vi "Periodic Tasks.vi"(8 "error in":errorcluster) -> ()   [LabVIEW 2018]
doc: "This VI runs in parallel to other tasks. It can contain as many user-defined periodic loops as you need. These can carry out PID or other sorts of timed response."
uses:
  <vilib>/Rock Robotics/WPI/Utilities/WPI_GetSetVariantRefNum.vi
  Robot Global Data.vi
panel:
  in  "PID Constants":T1={"proportional gain (Kc)"=1.0, "integral time (Ti, min)"=0.01, "derivative time (Td, min)"=0.0} {"derivative time (Td, min)" format="%.3f"; "integral time (Ti, min)" format="%.3f"; "proportional gain (Kc)" format="%.3f"}
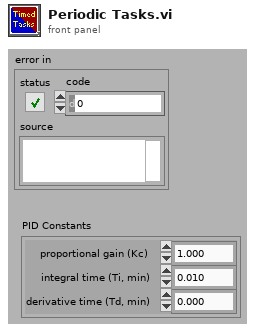
[diagram p1: front panel]
types:
  T1 = cluster{"proportional gain (Kc)":dbl, "integral time (Ti, min)":dbl, "derivative time (Td, min)":dbl}
  T2 = typedef "WPI_MotorControlDeviceRef.ctl" = cluster{"DeviceStatus":errorcluster, "Type":T3, "PWM":cluster{"PWM Channel":T4, "DeadBand":T5}, "CAN":cluster{"Device Number":u8, "SetOutput VI Ref":variant, "GetOutput VI Ref":variant, "Enable VI Ref":variant, "Disable VI Ref":variant, "Data":variant}, "Invert":bool, "DIO PWM":cluster{"PWM \"Enable\" Channel":T4, "DIOChannel":T6, "PWM Rate":dbl}}
  T3 = typedef "WPI_MotorControlType.ctl" = enum16{"PWM", "CAN", "DIO PWM"}
  T4 = typedef "FPGA_DIOPWMChannel.ctl" = enum8{"PWM 0", "PWM 1", "PWM 2", "PWM 3", "PWM 4", "PWM 5", "PWM 6", "PWM 7", "PWM 8", "PWM 9", "PWM MXP 0", "PWM MXP 1", "PWM MXP 2", "PWM MXP 3", "PWM MXP 4", "PWM MXP 5", "PWM MXP 6", "PWM MXP 7", "PWM MXP 8", "PWM MXP 9", "Invalid"}
  T5 = typedef "WPI_PWMDeadband.ctl" = cluster{"Name":string, "maxPositivePwm":i32, "minPositivePwm":i32, "centerPwm":i32, "maxNegativePwm":i32, "minNegativePwm":i32, "angularRange":u16}
  T6 = typedef "FPGA_DIOChannel.ctl" = enum8{"DIO 0", "DIO 1", "DIO 2", "DIO 3", "DIO 4", "DIO 5", "DIO 6", "DIO 7", "DIO 8", "DIO 9", "DIO MXP 0", "DIO MXP 1", "DIO MXP 2", "DIO MXP 3", "DIO MXP 4", "DIO MXP 5", "DIO MXP 6", "DIO MXP 7", "DIO MXP 8", "DIO MXP 9", "DIO MXP 10", "DIO MXP 11", "DIO MXP 12", "DIO MXP 13", "DIO MXP 14", "DIO MXP 15", "SPI Port CS1", "SPI Port CS2", "SPI Port CS3", "SPI Port MISO", "SPI Port MOSI", "Invalid"}
  T7 = typedef "WPI_JoystickDevRef.ctl" = cluster{"Device":T8}
  T8 = typedef "WPI_JoystickDeviceEnum.ctl" = enum16{"USB 0", "USB 1", "USB 2", "USB 3", "USB 4", "USB 5"}
  T9 = typedef "WPI_SolenoidDevRef.ctl" = cluster{"DevStatus":errorcluster, "Pneumatics Control Module":u8, "Forward Solenoid Channel":T10, "Reverse Solenoid Channel":T10}
  T10 = typedef "WPI_SolenoidChannel.ctl" = enum8{"Solenoid 0", "Solenoid 1", "Solenoid 2", "Solenoid 3", "Solenoid 4", "Solenoid 5", "Solenoid 6", "Solenoid 7", "Invalid"}
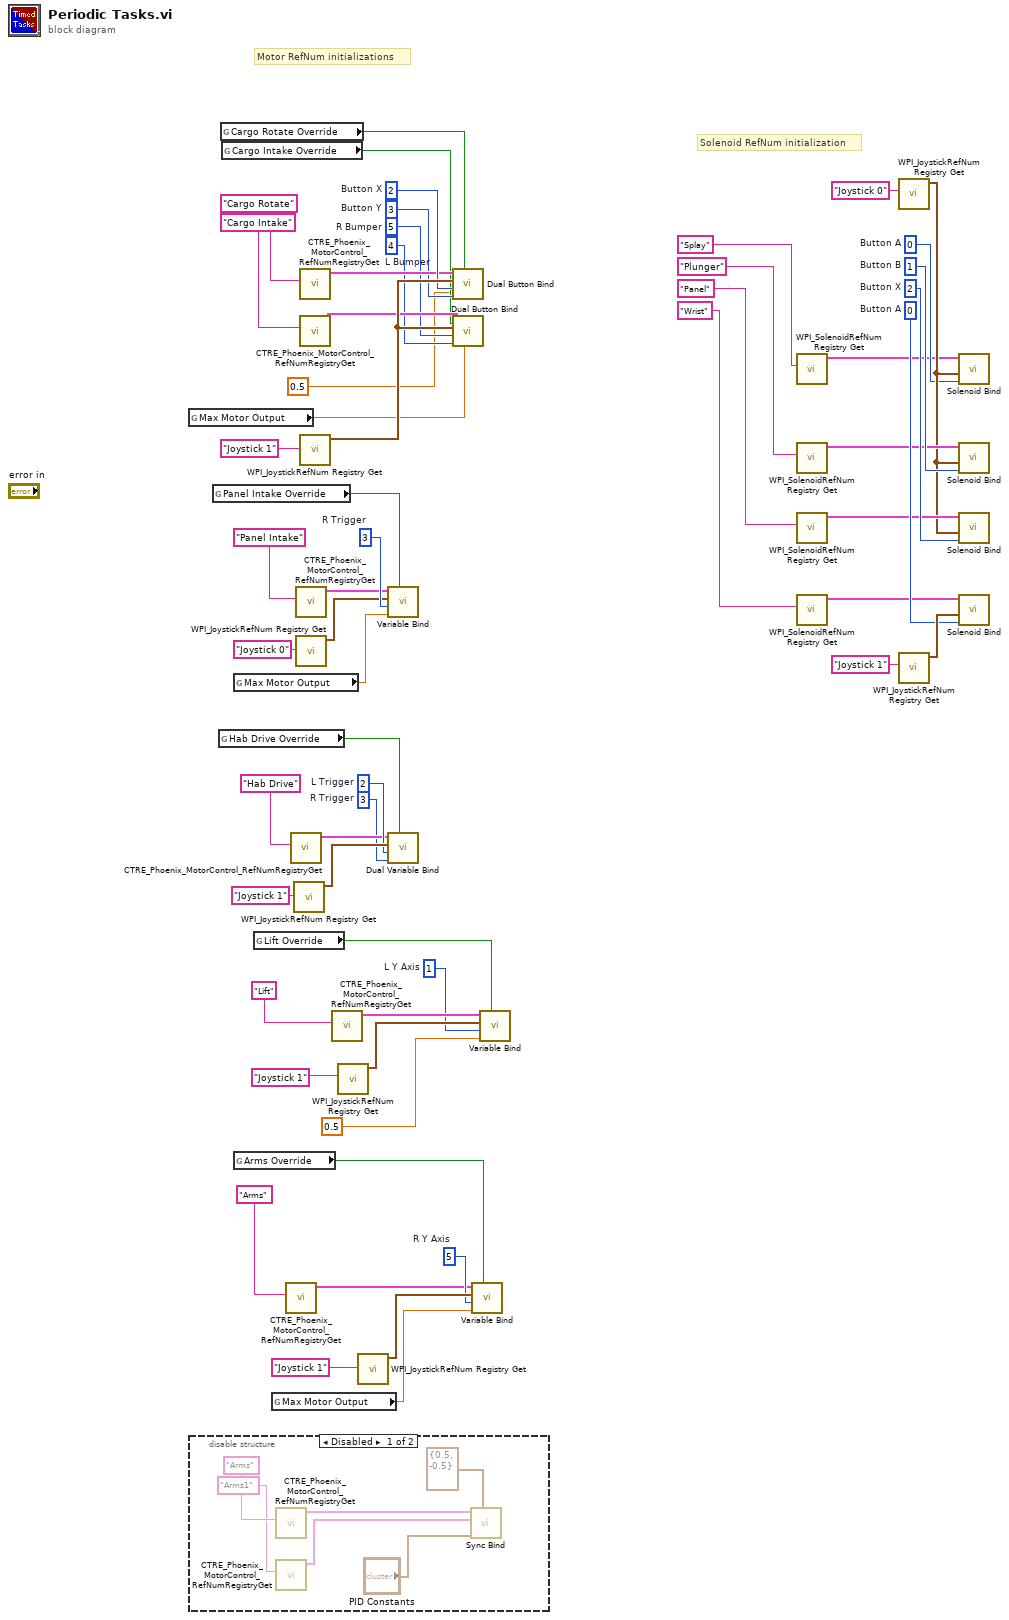
[diagram p0: block diagram]
diagram:
  w32 = 0  # Button A
  w34 = 2  # Button X
  w33 = 1  # Button B
  w27 = 0  # Button A
  w56 = 5  # R Y Axis
  w10 = 1  # L Y Axis
  w13 = 3  # R Trigger
  w50 = 2  # L Trigger
  w49 = 3  # R Trigger
  w14 = 4  # L Bumper
  w16 = 3  # Button Y
  w15 = 5  # R Bumper
  w43 = 2  # Button X
  # "Solenoid RefNum initialization"
  # "Motor RefNum initializations"
  n1 = global read "Robot Global Data.vi" "Max Motor Output"() -> (w2:dbl)
  n2 = disable-structure shown="Disabled" {
    frame Disabled {
      n3 = call <vilib>:"CTRE_Phoenix_MotorControl_RefNumRegistryGet.vi"("refnum name"="Arms") -> ("PhoenixMotorControlDevRef"=w62:T2)  [unwired: 9 in, 1 out]
      n4 = call <vilib>:"CTRE_Phoenix_MotorControl_RefNumRegistryGet.vi"("refnum name"="Arms1") -> ("PhoenixMotorControlDevRef"=w61:T2)  [unwired: 9 in, 1 out]
      n5 = call "Sync Bind.vi"("output range"=cluster{"output high":dbl, "output low":dbl} {"output high"=0.5, "output low"=-0.5}, "PID Constants"="PID Constants", "SlaveDevRef"=w61, "MasterDevRef"=w62) -> ()  [unwired: 8 in]
    }
    frame Enabled {
    }
  }
  n6 = global read "Robot Global Data.vi" "Panel Intake Override"() -> (w7:bool)
  n7 = global read "Robot Global Data.vi" "Hab Drive Override"() -> (w6:bool)
  n8 = global read "Robot Global Data.vi" "Cargo Rotate Override"() -> (w9:bool)
  n9 = global read "Robot Global Data.vi" "Cargo Intake Override"() -> (w8:bool)
  n10 = global read "Robot Global Data.vi" "Max Motor Output"() -> (w54:dbl)
  n11 = global read "Robot Global Data.vi" "Arms Override"() -> (w4:bool)
  n12 = global read "Robot Global Data.vi" "Lift Override"() -> (w5:bool)
  n13 = global read "Robot Global Data.vi" "Max Motor Output"() -> (w55:dbl)
  n14 = call <vilib>:"CTRE_Phoenix_MotorControl_RefNumRegistryGet.vi"("refnum name"="Arms") -> ("PhoenixMotorControlDevRef"=w20:T2)  [unwired: 9 in, 1 out]
  n15 = call <vilib>:"CTRE_Phoenix_MotorControl_RefNumRegistryGet.vi"("refnum name"="Hab Drive") -> ("PhoenixMotorControlDevRef"=w19:T2)  [unwired: 9 in, 1 out]
  n16 = call <vilib>:"WPI_JoystickRefNum Registry Get.vi"("refnum name"="Joystick 1") -> ("JoystickDevRef"=w52:T7)  [unwired: 9 in, 1 out]
  n17 = call <vilib>:"CTRE_Phoenix_MotorControl_RefNumRegistryGet.vi"("refnum name"="Panel Intake") -> ("PhoenixMotorControlDevRef"=w47:T2)  [unwired: 9 in, 1 out]
  n18 = call <vilib>:"WPI_JoystickRefNum Registry Get.vi"("refnum name"="Joystick 0") -> ("JoystickDevRef"=w48:T7)  [unwired: 9 in, 1 out]
  n19 = call <vilib>:"CTRE_Phoenix_MotorControl_RefNumRegistryGet.vi"("refnum name"="Cargo Rotate") -> ("PhoenixMotorControlDevRef"=w18:T2)  [unwired: 9 in, 1 out]
  n20 = call <vilib>:"CTRE_Phoenix_MotorControl_RefNumRegistryGet.vi"("refnum name"="Cargo Intake") -> ("PhoenixMotorControlDevRef"=w17:T2)  [unwired: 9 in, 1 out]
  n21 = call <vilib>:"WPI_JoystickRefNum Registry Get.vi"("refnum name"="Joystick 1") -> ("JoystickDevRef"=w45:T7)  [unwired: 9 in, 1 out]
  n22 = call <vilib>:"CTRE_Phoenix_MotorControl_RefNumRegistryGet.vi"("refnum name"="Lift") -> ("PhoenixMotorControlDevRef"=w12:T2)  [unwired: 9 in, 1 out]
  n23 = call <vilib>:"WPI_JoystickRefNum Registry Get.vi"("refnum name"="Joystick 1") -> ("JoystickDevRef"=w11:T7)  [unwired: 9 in, 1 out]
  n24 = call <vilib>:"WPI_JoystickRefNum Registry Get.vi"("refnum name"="Joystick 1") -> ("JoystickDevRef"=w57:T7)  [unwired: 9 in, 1 out]
  n25 = call "Variable Bind.vi"("Override"=w7, "Ouput"=w54, "Axis ID"=w49, "JoystickDevRef"=w48, "PhoenixMotorControlDevRef"=w47) -> ()  [unwired: 6 in, 1 out]
  n26 = call "Dual Variable Bind.vi"("Override"=w6, "Reverse ID"=w13, "Forward ID"=w50, "JoystickDevRef"=w52, "PhoenixMotorControlDevRef"=w19) -> ()  [unwired: 6 in, 1 out]
  n27 = call "Dual Button Bind.vi"("Output"=0.5, "Override"=w9, "Reverse ID"=w16, "Forward ID"=w43, "JoystickDevRef"=w45, "PhoenixMotorControlDevRef"=w18) -> ()  [unwired: 5 in, 1 out]
  n28 = call "Dual Button Bind.vi"("Output"=w2, "Override"=w8, "Reverse ID"=w14, "Forward ID"=w15, "JoystickDevRef"=w45, "PhoenixMotorControlDevRef"=w17) -> ()  [unwired: 5 in, 1 out]
  n29 = call "Variable Bind.vi"("Override"=w4, "Ouput"=w55, "Axis ID"=w56, "JoystickDevRef"=w57, "PhoenixMotorControlDevRef"=w20) -> ()  [unwired: 6 in, 1 out]
  n30 = call "Variable Bind.vi"("Override"=w5, "Ouput"=0.5, "Axis ID"=w10, "JoystickDevRef"=w11, "PhoenixMotorControlDevRef"=w12) -> ()  [unwired: 6 in, 1 out]
  n31 = call <vilib>:"WPI_SolenoidRefNum Registry Get.vi"("refnum name"="Splay") -> ("SolenoidDevRef"=w26:T9)  [unwired: 9 in, 1 out]
  n32 = call <vilib>:"WPI_SolenoidRefNum Registry Get.vi"("refnum name"="Plunger") -> ("SolenoidDevRef"=w29:T9)  [unwired: 9 in, 1 out]
  n33 = call <vilib>:"WPI_SolenoidRefNum Registry Get.vi"("refnum name"="Panel") -> ("SolenoidDevRef"=w30:T9)  [unwired: 9 in, 1 out]
  n34 = call <vilib>:"WPI_SolenoidRefNum Registry Get.vi"("refnum name"="Wrist") -> ("SolenoidDevRef"=w31:T9)  [unwired: 9 in, 1 out]
  n35 = call <vilib>:"WPI_JoystickRefNum Registry Get.vi"("refnum name"="Joystick 0") -> ("JoystickDevRef"=w28:T7)  [unwired: 9 in, 1 out]
  n36 = call <vilib>:"WPI_JoystickRefNum Registry Get.vi"("refnum name"="Joystick 1") -> ("JoystickDevRef"=w36:T7)  [unwired: 9 in, 1 out]
  n37 = call "Solenoid Bind.vi"("Button ID"=w27, "JoystickDevRef"=w28, "SolenoidDevRef"=w26) -> ()  [unwired: 9 in]
  n38 = call "Solenoid Bind.vi"("Button ID"=w33, "JoystickDevRef"=w28, "SolenoidDevRef"=w29) -> ()  [unwired: 9 in]
  n39 = call "Solenoid Bind.vi"("Button ID"=w34, "JoystickDevRef"=w28, "SolenoidDevRef"=w30) -> ()  [unwired: 9 in]
  n40 = call "Solenoid Bind.vi"("Button ID"=w32, "JoystickDevRef"=w36, "SolenoidDevRef"=w31) -> ()  [unwired: 9 in]
